vi "Format Control Packet.vi"(9 "Payload":u8[](array[numeric]) format="%08b", 10 "Variable Header":u8[](array[numeric]) format="%08b", 11 "Fixed Header":u8 format="%08b") -> (3 "Control Packet":u8[](array[numeric]) format="%08b")   [LabVIEW 2013]
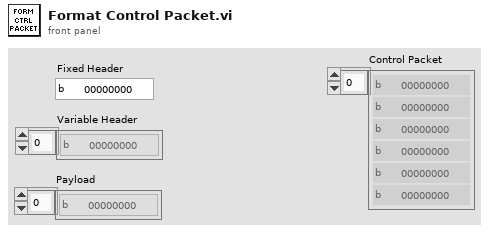
[diagram p1: front panel]
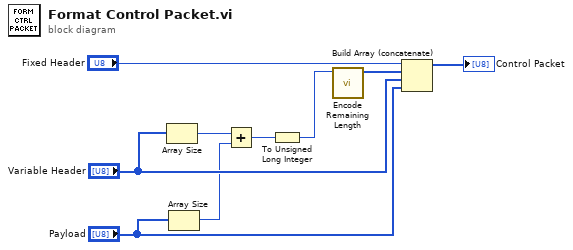
[diagram p0: block diagram]
diagram:
  n1 = Array Size(array="Variable Header") -> (size(s)=w4:i32)
  n2 = Array Size(array="Payload") -> (size(s)=w5:i32)
  n3 = Add(x=w4, y=w5) -> (x+y=w3:i32)
  n4 = To Unsigned Long Integer(number=w3) -> (unsigned 32bit integer=w2:u32)
  n5 = call "Encode Remaining Length.vi"("Remaining Length (bytes)"=w2) -> ("Encoded Remaining Length"=w1:u8[])  [unwired: 9 in, 1 out]
  n6 = Build Array (concatenate)("Fixed Header", w1, "Variable Header", "Payload") -> (→"Control Packet":u8[])
